vi "sitios.vi"() -> ()   [LabVIEW 2010]
uses:
  <vilib>/addons/PixeLINK/Low Level Functions/CAMERA_FEATURES.llb/TDPU-CameraFeatures-PixelFormat.ctl
  <vilib>/Utility/error.llb/DialogType.ctl
  <vilib>/Utility/file.llb/Write To Spreadsheet File (DBL).vi
  <vilib>/vision/NI_Vision_Development_Module.lvlib
panel:
  out "Paso final":dbl
  in  "Veces":u16=10
  in  "Paso inicial":dbl=0.25
  in  "Valor Final":dbl=10.0
  out "In Range?":bool
  in  "tiempo de espera (ms)":u32=5000
  out "Paso actual":i32
  in  "nombre archivo":string="paso"
  out "Cantidad de pasos":u32=16
  in  "base path":path=path "C:/Users/veloz/Documents/tesis/codigos/Matlab/archivos"
  in  "Tamaño entre pasos":dbl=0.25
  out "Veces Realizado":i32
  in  "Imagenes":i32=5
  in  "tiempo entre pasos (ms)":dbl=2000.0
  out "Tamaño del paso":dbl=4.0
  in  "Valor Inicial":dbl=-10.0
  out "Array":T1[](array[plugin-control])
  in  "Start":bool
  out "Image OUT":T1(plugin-control)
  out "new file path":path
  in  "stop":bool
  out "Imagenes tomadas":i32
  in  "Camara Parameters":T3 {"Pixel Format" items=["PIXEL_FORMAT_MONO8", "PIXEL_FORMAT_MONO16", "PIXEL_FORMAT_YUV422", "PIXEL_FORMAT_BAYER8_GRBG", "PIXEL_FORMAT_BAYER16_GRBG", "PIXEL_FORMAT_RGB24", "PIXEL_FORMAT_RGB48", "PIXEL_FORMAT_BAYER8_RGGB", "PIXEL_FORMAT_BAYER8_GBRG ", "PIXEL_FORMAT_BAYER8_BGGR ", "PIXEL_FORMAT_BAYER16_RGGB ", "PIXEL_FORMAT_BAYER16_GBRG", "PIXEL_FORMAT_BAYER16_BGGR", "PIXEL_FORMAT_RGB32"]}
  in  "Selector":u16(ring) items=["776002034"]
  in  "Streeam?":bool
  in  "DAQ Controls":T4={"Minimum Value"=-10.0, "Maximum Value"=10.0, "Physical Channel"="Dev1/ao0", "DAQ Fs (S/s)"=10000.0} {"Minimum Value" min=-10.0 max=0.0; "Maximum Value" min=0.0 max=10.0}
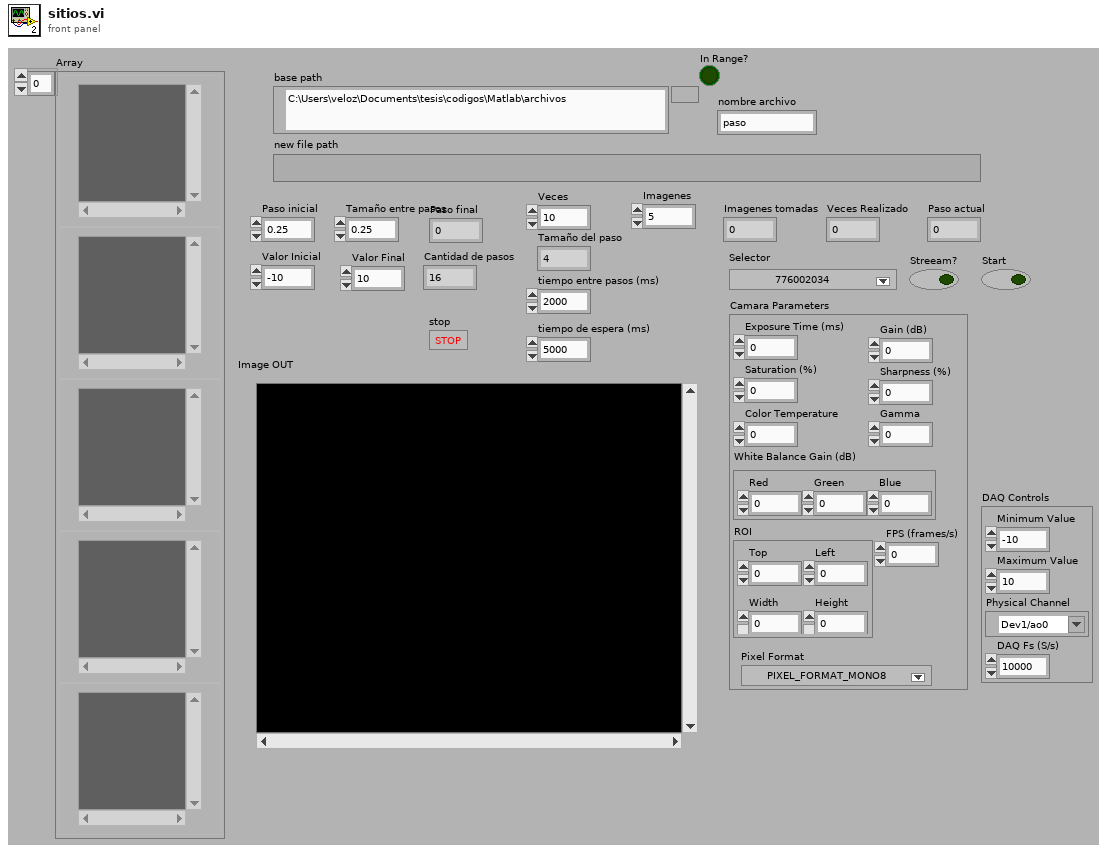
[diagram p1: front panel]
types:
  T1 = typedef "IMAQ Image.ctl" = refnum<image>
  T2 = typedef "TDPU-CameraFeatures-PixelFormat.ctl" = u16
  T3 = cluster{"Exposure Time (ms)":dbl, "Gain (dB)":dbl, "Saturation (%)":dbl, "Sharpness (%)":dbl, "Color Temperature":dbl, "ROI":cluster{"Top":i32, "Left":i32, "Width":i32, "Height":i32}, "White Balance Gain (dB)":cluster{"Red":dbl, "Green":dbl, "Blue":dbl}, "Gamma":dbl, "Pixel Format":T2, "FPS (frames/s)":i32}
  T4 = cluster{"Minimum Value":dbl, "Maximum Value":dbl, "Physical Channel":tag, "DAQ Fs (S/s)":dbl}
  T5 = cluster{"DAQ Fs (S/s)":dbl, "task":refnum<k21>, "error":errorcluster, "Min Value":dbl, "Max Value":dbl}
  T6 = cluster{"hCamera":u32, "Error":errorcluster, "uSerialNumber OUT":u32}
  T7 = cluster{"hCamera":u32, "Error":errorcluster, "uSerialNumber":u32}
  T8 = cluster{"DAQ Limits":cluster{"max":dbl, "min":dbl}, "Control Limits":cluster{"max":dbl, "min":dbl}}
  T9 = typedef "Image Type" = u32
  T10 = typedef "DialogType.ctl" = u16
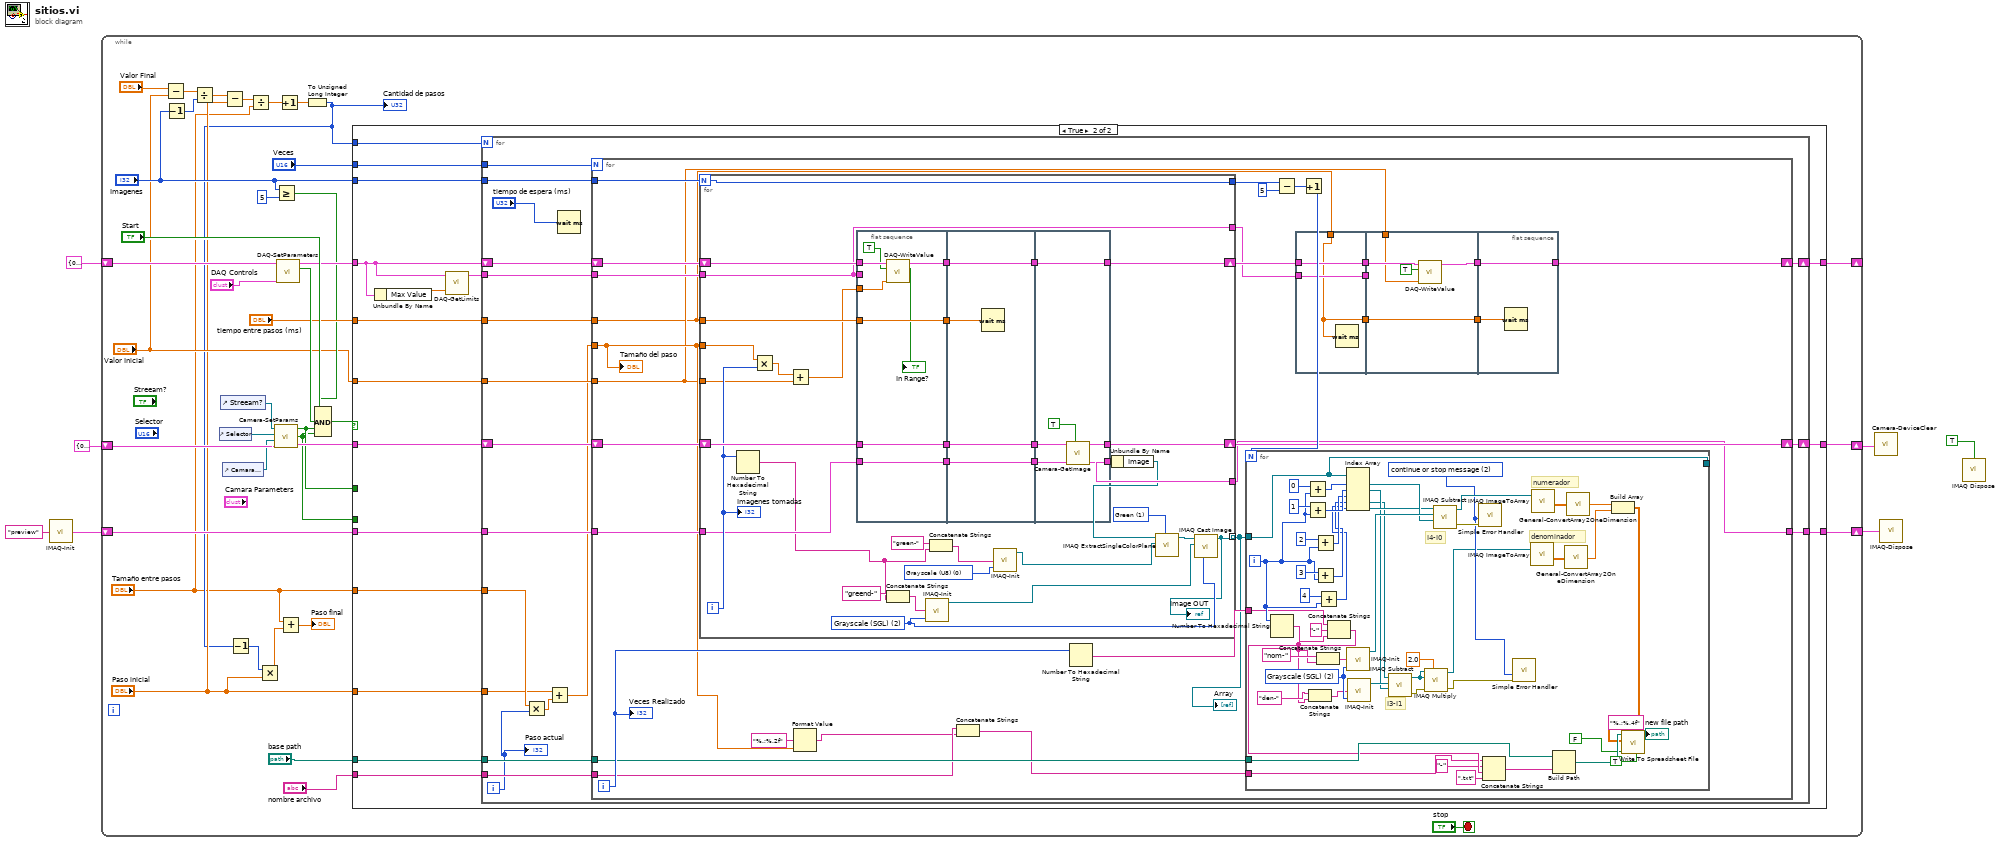
[diagram p0: block diagram]
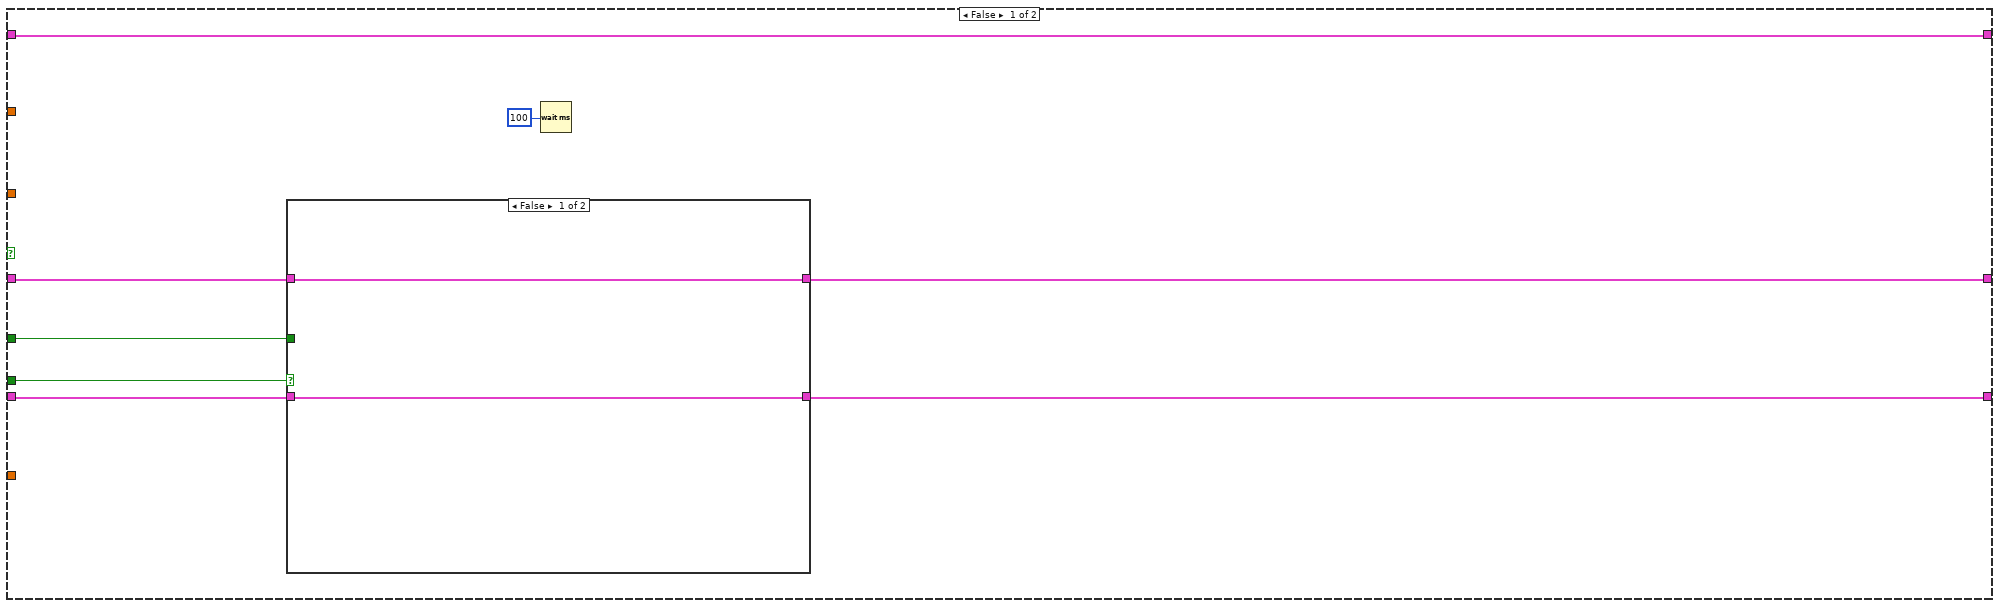
[diagram p2: hidden frame]
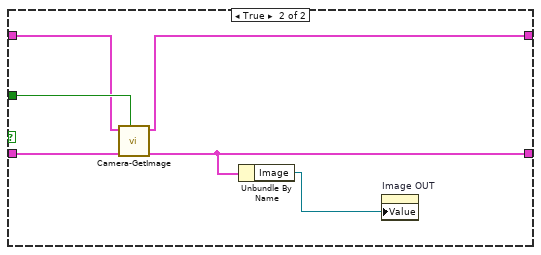
[diagram p3: hidden frame]
diagram:
  n1 = call "IMAQ-Init.vi"("Image Name"="preview") -> ("Image Device OUT"=w3:cluster{"Image":T1, "errorImage":errorcluster})  [unwired: 2 in, 2 out]
  n2 = while {
    shift-right: [w34] -> w1
    shift-left: T6 {"hCamera"=0, "Error"={"status"=FALSE, "code"=0, "source"=""}, "uSerialNumber OUT"=0} ("Camera Device  IN") -> [w41]
    shift-right: [w35] -> _
    shift-left: T5 {"DAQ Fs (S/s)"=0.0, "task"="", "error"={"status"=FALSE, "code"=0, "source"=""}, "Min Value"=0.0, "Max Value"=0.0} ("DAQ Device OUT") -> [w36]
    shift-right: [w24] -> w2
    shift-left: w3 -> [w26]
    stop <- "stop" stop-if-true
    n3 = Subtract(x="Valor Final", y="Valor Inicial") -> (x-y=w20:dbl)
    n4 = Decrement(x="Imagenes") -> (x-1=w21:i32)
    n5 = Divide(x=w20, y=w21) -> (x/y=w19:dbl)
    n6 = control-ref of="Selector"() -> (w45:refnum<vi>)
    n7 = control-ref of="Streeam?"() -> (w44:refnum<vi>)
    n8 = control-ref of="Camara Parameters"() -> (w43:refnum<vi>)
    n9 = Subtract(x=w19, y="Paso inicial") -> (x-y=w18:dbl)
    n10 = Divide(x=w18, y="Tamaño entre pasos") -> (x/y=w17:dbl)
    n11 = call "Camera-SetParams.vi"("Camera Device  IN"=w41, "Camera Parameters"=w43, "Selector"=w45, "Stream?"=w44) -> ("Camera Device OUT"=w42:T7, "Funciona?"=w23:bool, "Stream? OUT"=w25:bool)
    n12 = Greater Or Equal?(x="Imagenes", y=5) -> (x >= y?=w31:bool)
    n13 = call "DAQ-SetParameters.vi"("DAQ Controls"="DAQ Controls", "DAQ Device IN"=w36) -> ("En Funcionamiento?"=w39:bool, "DAQ Device OUT"=w37:T5)  [unwired: 4 in]
    n14 = Increment(x=w17) -> (x+1=w22:dbl)
    n15 = To Unsigned Long Integer(number=w22) -> (unsigned 32bit integer=w11:u32)
    "Cantidad de pasos" <- w11
    n16 = Decrement(x=w11) -> (x-1=w12:u32)
    n17 = Multiply(x=w12, y="Paso inicial") -> (x*y=w10:dbl)
    n18 = Add(x="Tamaño entre pasos", y=w10) -> (x+y=→"Paso final":dbl)
    n19 = Compound Arithmetic op=AND(w31, "Start", w39, w25, w23) -> (w40:bool)
    n20 = case shown="True" w40 {
      tunnel: w42 -> [w50 w79]
      tunnel: [w49 w71] -> w34
      tunnel: w37 -> [w53 w72]
      tunnel: [w53 w78] -> w35
      tunnel: "tiempo entre pasos (ms)" -> [_ w74]
      tunnel: "Imagenes" -> [_ w77]
      tunnel: "Valor Inicial" -> [_ w73]
      tunnel: "Veces" -> [_ w70]
      tunnel: "base path" -> [_ w69]
      tunnel: "nombre archivo" -> [_ w68]
      tunnel: w26 -> [w52 w67]
      tunnel: w25 -> [w51 _]
      tunnel: [w48 w66] -> w24
      tunnel: w23 -> [w47 _]
      tunnel: "Tamaño entre pasos" -> [_ w65]
      tunnel: w11 -> [_ w64]
      tunnel: "Paso inicial" -> [_ w63]
      frame False {
        n21 = case shown="False" w47 {
          tunnel: w52 -> [w55 w62]
          tunnel: w51 -> [_ w61]
          tunnel: w50 -> [w56 w60]
          tunnel: [w56 w59] -> w49
          tunnel: [w55 w58] -> w48
          frame False {
          }
          frame True {
            n22 = call "Camera-GetImage.vi"("Streeam"=w61, "Image Device IN"=w62, "Camera Device IN"=w60) -> ("Image Device OUT"=w58:cluster{"Image":T1, "errorImage":errorcluster}, "Camera Device OUT"=w59:T7)  [unwired: 4 in]
            n23 = Unbundle By Name(w58) -> ("Image"=w57:T1)
            n24 = property on="Image OUT" class="ImageControl"("Value"=w57) -> ()  [unwired: 2 in, 2 out]
          }
        }
        n25 = Wait (ms)(milliseconds to wait=u32 100) -> ()  [unwired: 1 out]
      }
      frame True {
        n26 = Unbundle By Name(w72) -> ("Max Value"=w76:dbl)
        n27 = call "DAQ-GetLimits.vi"("Amplitud"=w76, "DAQ Device IN"=w72) -> ("Limites"=w75:T8)  [unwired: 3 in]
        n28 = for {
          N: w64 -> [_]
          tunnel: w77 -> [w96]
          tunnel: w75 -> [w95]
          tunnel: w74 -> [w94]
          tunnel: w73 -> [w93]
          tunnel: w70 -> [w90]
          tunnel: w69 -> [w89]
          tunnel: w68 -> [w88]
          tunnel: w67 -> [w87]
          tunnel: [w86] -> w66
          shift-right: [w91] -> w71
          shift-left: w79 -> [w98]
          shift-right: [w97] -> w78
          shift-left: w72 -> [w92]
          tunnel: w65 -> [w85]
          tunnel: w63 -> [w80]
          i -> [w82]
          n29 = Multiply(x=w85, y=w82) -> (x*y=w81:dbl)
          n30 = Add(x=w80, y=w81) -> (x+y=w83:dbl)
          n31 = Wait (ms)(milliseconds to wait="tiempo de espera (ms)") -> ()  [unwired: 1 out]
          n32 = for {
            N: w90 -> [_]
            tunnel: w96 -> [w127]
            tunnel: w95 -> [w126]
            tunnel: w94 -> [w101]
            tunnel: w83 -> [w111]
            tunnel: w93 -> [w105]
            shift-right: [w107] -> w97
            shift-left: w92 -> [w120]
            shift-right: [w119] -> w91
            shift-left: w98 -> [w128]
            tunnel: w89 -> [w117]
            tunnel: w88 -> [w113]
            tunnel: w87 -> [w116]
            tunnel: [w115] -> w86
            i -> [w118]
            n33 = for {
              N: w127 -> [w204]
              tunnel: w126 -> [w189]
              tunnel: w101 -> [w211]
              tunnel: w111 -> [w209]
              tunnel: w105 -> [w207]
              tunnel: [w190] -> w114 mode=indexing
              tunnel: [w204] -> w125
              shift-right: [w221] -> w108
              shift-left: w120 -> [w222]
              shift-right: [w215] -> w119
              shift-left: w128 -> [w218]
              tunnel: w116 -> [w201]
              tunnel: [w200] -> w115
              tunnel: [w189] -> w106
              i -> [w210]
              w195 = T9 2 items=["Grayscale (U8)", "Grayscale (I16)", "Grayscale (SGL)", "Complex (CSG)", "RGB (U32)", "HSL (U32)", "RGB (U64)", "Grayscale (U16)"] ("Image Type")
              w199 = 1 items=["Red", "Green", "Blue", "Hue", "Saturation", "Luminance", "Value", "Intensity"] ("Color Plane")
              w202 = T9 0 items=["Grayscale (U8)", "Grayscale (I16)", "Grayscale (SGL)", "Complex (CSG)", "RGB (U32)", "HSL (U32)", "RGB (U64)", "Grayscale (U16)"] ("Image Type")
              n34 = Number To Hexadecimal String(2:w210) -> (0:w193:string)  [unwired: 1 in]
              n35 = Multiply(x=w209, y=w210) -> (x*y=w206:dbl)
              n36 = Add(x=w206, y=w207) -> (x+y=w208:dbl)
              n37 = flat-sequence {
                tunnel: w189 -> [_]
                tunnel: w222 -> [w230]
                tunnel: [w229] -> w220
                tunnel: w218 -> [w228]
                tunnel: [w228] -> w216
                tunnel: [w227] -> w213
                tunnel: w201 -> [w227]
                tunnel: [w226] -> w212
                tunnel: w211 -> [w226]
                tunnel: w208 -> [w224]
                tunnel: w220 -> [w234]
                tunnel: [w234] -> w219
                tunnel: [w233] -> w217
                tunnel: w216 -> [w233]
                tunnel: [w232] -> w214
                tunnel: w213 -> [w232]
                tunnel: w212 -> [w231]
                tunnel: [w240] -> w221
                tunnel: w219 -> [w240]
                tunnel: w217 -> [w239]
                tunnel: [w238] -> w215
                tunnel: w214 -> [w237]
                tunnel: [w236] -> w200
                frame #0 {
                  n38 = call "DAQ-WriteValue.vi"("Input"=w224, "DAQ?"=TRUE, "DAQ Device IN"=w230) -> ("In Range?"=→"In Range?":bool, "DAQ Device OUT"=w229:T5)  [unwired: 5 in]
                }
                frame #1 {
                  n39 = Wait (ms)(milliseconds to wait=w231) -> ()  [unwired: 1 out]
                }
                frame #2 {
                  n40 = call "Camera-GetImage.vi"("Streeam"=TRUE, "Image Device IN"=w237, "Camera Device IN"=w239) -> ("Image Device OUT"=w236:cluster{"Image":T1, "errorImage":errorcluster}, "Camera Device OUT"=w238:T7)  [unwired: 4 in]
                }
              }
              n41 = Concatenate Strings("greend-" ("string"), w193) -> (w192:string)
              n42 = call "IMAQ-Init.vi"("Image Type"=w195, "Image Name"=w192) -> ("Image OUT"=w196:T1)  [unwired: 1 in, 2 out]
              n43 = Concatenate Strings("green-" ("string"), w193) -> (w203:string)
              n44 = call "IMAQ-Init.vi"("Image Type"=w202, "Image Name"=w203) -> ("Image OUT"=w198:T1)  [unwired: 1 in, 2 out]
              n45 = Unbundle By Name(w200) -> ("Image"=w191:T1)
              n46 = call "IMAQ ExtractSingleColorPlane"("Color Plane"=w199, "Image Dst"=w198, "Image Src"=w191) -> ("Image Dst Out"=w197:T1)  [unwired: 7 in, 1 out]
              n47 = call "IMAQ Cast Image"("Image Type"=w195, "Image Dst"=w196, "Image Src"=w197) -> ("Image Dst Out"=w190:T1)  [unwired: 7 in, 1 out]
              "Image OUT" <- w190
              "Imagenes tomadas" <- w210
            }
            "Array" <- w114
            n48 = Format Value(format string="%.;%.2f", value (0)=w111) -> (output string=w109:string)  [unwired: 1 in]
            n49 = Concatenate Strings(w113, w109) -> (w112:string)
            n50 = Number To Hexadecimal String(2:w118) -> (0:w121:string)  [unwired: 1 in]
            n51 = Subtract(x=w125, y=5) -> (x-y=w123:i32)
            n52 = flat-sequence {
              tunnel: w106 -> [w130]
              tunnel: w108 -> [w131]
              tunnel: [w131] -> w104
              tunnel: [w130] -> w103
              tunnel: w101 -> [w129]
              tunnel: [w129] -> w99
              tunnel: w105 -> [w133]
              tunnel: w104 -> [w136]
              tunnel: w103 -> [_]
              tunnel: [w135] -> w102
              tunnel: [w132] -> w100
              tunnel: w99 -> [w132]
              tunnel: [w138] -> w107
              tunnel: w102 -> [w138]
              tunnel: w100 -> [w137]
              frame #0 {
                n53 = Wait (ms)(milliseconds to wait=w129) -> ()  [unwired: 1 out]
              }
              frame #1 {
                n54 = call "DAQ-WriteValue.vi"("Input"=w133, "DAQ?"=TRUE, "DAQ Device IN"=w136) -> ("DAQ Device OUT"=w135:T5)  [unwired: 5 in, 1 out]
              }
              frame #2 {
                n55 = Wait (ms)(milliseconds to wait=w137) -> ()  [unwired: 1 out]
              }
            }
            n56 = Increment(x=w123) -> (x+1=w122:i32)
            n57 = for {
              N: w122 -> [_]
              tunnel: w114 -> [w171]
              tunnel: [w171] -> _
              tunnel: w121 -> [w167]
              tunnel: w117 -> [w165]
              tunnel: w112 -> [w156]
              i -> [w170]
              w148 = T10 2 items=["no dialog", "OK message", "continue or stop message", "OK message + warnings", "continue/stop + warnings"] ("type of dialog (OK msg:1)")
              w155 = T9 2 items=["Grayscale (U8)", "Grayscale (I16)", "Grayscale (SGL)", "Complex (CSG)", "RGB (U32)", "HSL (U32)", "RGB (U64)", "Grayscale (U16)"] ("Image Type")
              # "I3-I1"
              # "I4-I0"
              # "denominador"
              # "numerador"
              n58 = Number To Hexadecimal String(2:w170) -> (0:w168:string)  [unwired: 1 in]
              n59 = Add(x=0, y=w170) -> (x+y=w180:i32)
              n60 = Add(x=1, y=w170) -> (x+y=w179:i32)
              n61 = Add(x=2, y=w170) -> (x+y=w178:i32)
              n62 = Add(x=3, y=w170) -> (x+y=w177:i32)
              n63 = Add(x=4, y=w170) -> (x+y=w176:i32)
              n64 = Concatenate Strings(w167, "-" ("string"), w168) -> (w163:string)
              n65 = Concatenate Strings("den-" ("Image Name"), w163) -> (w141:string)
              n66 = Concatenate Strings("nom-" ("Image Name"), w163) -> (w183:string)
              n67 = Index Array(array=w171, index #1=w180, index #2=w179, index #3=w178, index #4=w177, index #5=w176) -> (element #1=w154:T1, element #2=w152:T1, element #4=w151:T1, element #5=w153:T1)  [unwired: 1 out]
              n68 = call "IMAQ-Init.vi"("Image Type"=w155, "Image Name"=w183) -> ("Image OUT"=w172:T1)  [unwired: 1 in, 2 out]
              n69 = call "IMAQ-Init.vi"("Image Type"=w155, "Image Name"=w141) -> ("Image OUT"=w174:T1)  [unwired: 1 in, 2 out]
              n70 = call "IMAQ Subtract"("Image Src A"=w151, "Image Dst"=w174, "Image Src B"=w152) -> ("Image Dst Out"=w173:T1, "error out"=w150:errorcluster)  [unwired: 4 in]
              n71 = call "IMAQ Multiply"("Image Src A"=w173, "Constant"=sgl 2.0, "Image Dst"=w173, "error in (no error)"=w150) -> ("Image Dst Out"=w146:T1, "error out"=w139:errorcluster)  [unwired: 3 in]
              n72 = call "IMAQ Subtract"("Image Src A"=w153, "Image Dst"=w172, "Image Src B"=w154) -> ("Image Dst Out"=w166:T1, "error out"=w149:errorcluster)  [unwired: 4 in]
              n73 = call <vilib>:"Simple Error Handler.vi"("type of dialog (OK msg:1)"=w148, "error in (no error)"=w149) -> ()  [unwired: 3 in, 5 out]
              n74 = Concatenate Strings(w156, "-" ("string"), w163, ".txt" ("string")) -> (w164:string)
              n75 = call <vilib>:"Simple Error Handler.vi"("type of dialog (OK msg:1)"=w148, "error in (no error)"=w139) -> ()  [unwired: 3 in, 5 out]
              n76 = call "IMAQ ImageToArray"("Image"=w146) -> ("Image Pixels (Float)"=w143:sgl[][])  [unwired: 3 in, 4 out]
              n77 = call "IMAQ ImageToArray"("Image"=w166) -> ("Image Pixels (Float)"=w145:sgl[][])  [unwired: 3 in, 4 out]
              n78 = Build Path(base path=w165, name or relative path=w164) -> (appended path=w162:path)
              n79 = call "General-ConvertArray2OneDimension.vi"("Input Array"=w143) -> ("Output Array"=w142:dbl[])
              n80 = call "General-ConvertArray2OneDimension.vi"("Input Array"=w145) -> ("Output Array"=w144:dbl[])
              n81 = Build Array(w144, w142) -> (w161:dbl[][])
              n82 = call-poly <vilib>:"Write To Spreadsheet File.vi"("transpose? (no:F)"=TRUE, "format (%.3f)"="%.;%.4f", "append to file? (new file:F)"=FALSE, "2D data"=w161, "file path (dialog if empty)"=w162) -> ("new file path (Not A Path if cancelled)"=→"new file path":path)  [unwired: 3 in]
            }
            "Veces Realizado" <- w118
            "Tamaño del paso" <- w111
          }
          "Paso actual" <- w82
        }
      }
    }
  }
  n83 = call "Camera-DeviceClear.vi"("Camera Device OUT"=w1) -> ()
  n84 = call "IMAQ-Dispose.vi"("Image Device IN"=w2) -> ()
  n85 = call "IMAQ Dispose"("All Images? (No)"=TRUE) -> ()  [unwired: 5 in, 1 out]
